vi "OA_Wks-PutData.vi"(1 "Row 1":i32, 4 "error in (no error)":errorcluster, 5 "c1":i32, 6 "2d Data":sgl[][](array[numeric]) format="%0.3f", 7 "Origin.Worksheet":refnum<k7>) -> (0 "error out":errorcluster, 2 "PutData Result":bool=TRUE, 3 "Origin.Worksheet Out":refnum<k7>)   [LabVIEW 2010]
doc: "Send a 2D array to an Origin worksheet, starting from the c1 column. \nStarting row index (0 offset) is specified by Row 1, which you can set to -1 to append to existing data"
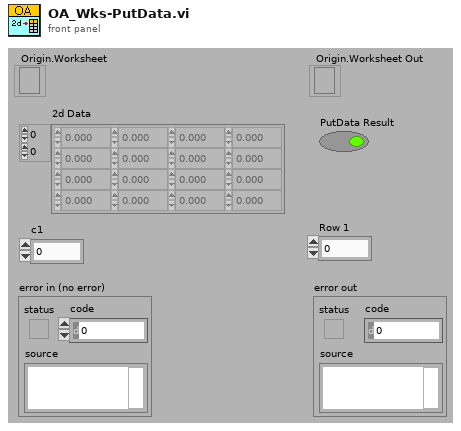
[diagram p1: front panel]
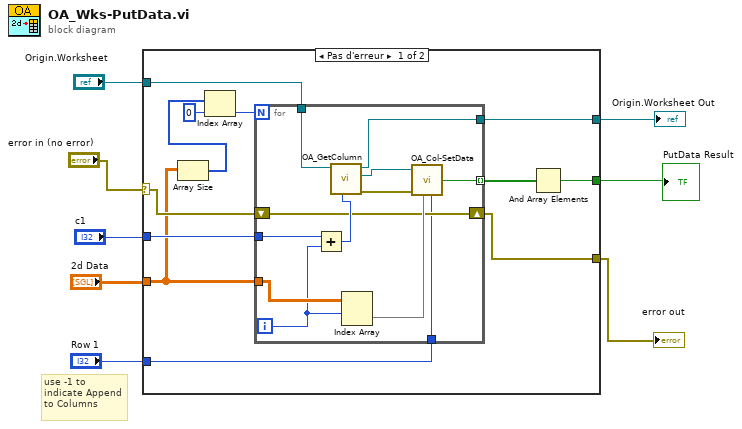
[diagram p0: block diagram]
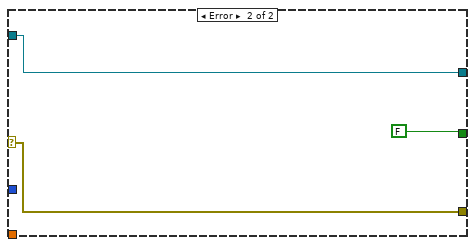
[diagram p2: hidden frame]
diagram:
  # "use -1 to indicate Append to Columns"
  n1 = case shown="Pas d'erreur" "error in (no error)" {
    selector: "error in (no error)" -> [w17 w34]
    tunnel: "2d Data" -> [w15 _]
    tunnel: "Origin.Worksheet" -> [w20 w33]
    tunnel: "c1" -> [w19 _]
    tunnel: [w16 w34] -> w4
    tunnel: [w18 w33] -> w3
    tunnel: [w10 FALSE] -> w2
    tunnel: "Row 1" -> [w9 _]
    frame No Error {
      n2 = Array Size(array=w15) -> (size(s)=w14:i32[])
      n3 = Index Array(array=w14, index=0) -> (element=w13:i32)
      n4 = for {
        N: w13 -> [_]
        tunnel: w20 -> [w32]
        tunnel: w19 -> [w31]
        tunnel: w15 -> [w30]
        tunnel: [w29] -> w18
        tunnel: [w24] -> w11 mode=indexing
        shift-right: [w22] -> w16
        shift-left: w17 -> [w22]
        tunnel: w9 -> [w21]
        i -> [w23]
        n5 = Add(x=w31, y=w23) -> (x+y=w26:i32)
        n6 = call <userlib>:"OA_GetColumn.vi"("Column Name/Index"=w26, "Origin.Worksheet"=w32) -> ("error out"=w27:errorcluster, "Origin.Column"=w28:refnum<k7>, "Origin.Worksheet"=w29:refnum<k7>)  [unwired: 7 in]
        n7 = Index Array(array=w30, index (row)=w23) -> (element=w25:sgl[])  [unwired: 1 in]
        n8 = call <userlib>:"OA_Col-SetData.vi"("Origin.Column"=w28, "error in (no error)"=w27, "data"=w25, "nOffset"=w21) -> ("SetData"=w24:bool)  [unwired: 3 in, 2 out]
      }
      n9 = And Array Elements(Boolean array=w11) -> (logical AND=w10:bool)
    }
    frame Error {
    }
  }
  "error out" <- w4
  "Origin.Worksheet Out" <- w3
  "PutData Result" <- w2
